vi "Dispose.vi"(8 "error in (no error)":errorcluster, 11 "LV-ORM in":refnum<class "LV-ORM.lvclass">) -> (0 "error out":errorcluster)   [LabVIEW 2018, in "LV-ORM.lvclass"]
uses:
  LV-ORM.lvclass
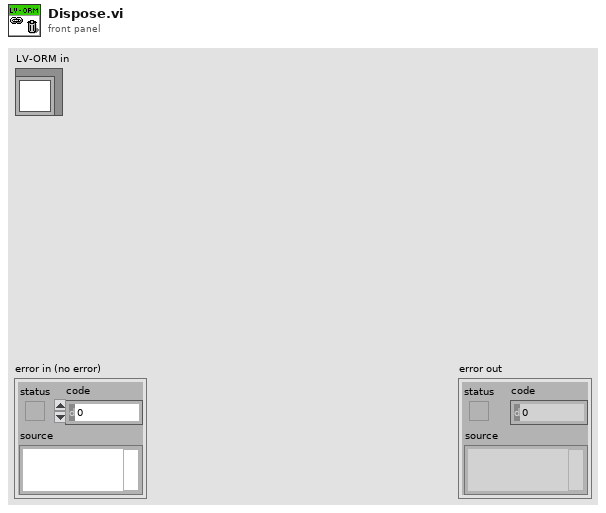
[diagram p1: front panel]
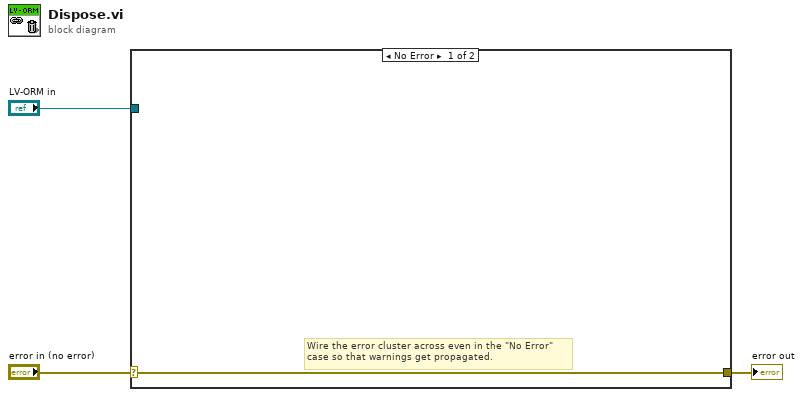
[diagram p0: block diagram]
diagram:
  n1 = case shown="No Error" "error in (no error)" {
    selector: "error in (no error)" -> [w4 w5]
    tunnel: [w4 w5] -> w2
    tunnel: "LV-ORM in" -> [_ _]
    frame No Error {
      # "Wire the error cluster across even in the \"No Error\"\ncase so that warnings get propagated."
    }
    frame Error {
    }
  }
  "error out" <- w2
